vi "CRYMultitone Sine.vi"(0 "Start Freq":dbl, 1 "Fs":dbl, 2 "Level In":dbl, 5 "Stop Freq":dbl, 7 "Step Number":i32, 9 "Resolution":u16, 11 "Cycles":dbl=1.0 max=3.0 step=1.0, 12 "Freq Rounding":bool, 13 "Rounding value":dbl, 14 "FAPS In":T1(array[cluster])) -> (4 "FAPS Out":T1(array[cluster]))   [LabVIEW 2013]
uses:
  CRYStimulus Global.vi
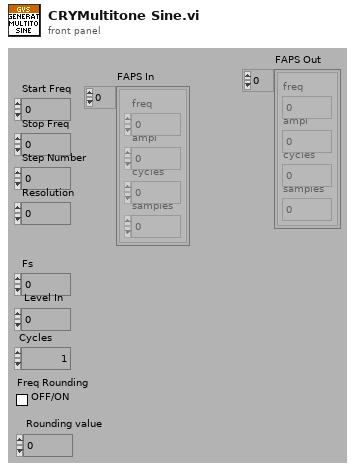
[diagram p1: front panel]
types:
  T1 = cluster{"freq":dbl, "ampl":dbl, "cycles":dbl, "samples":i32}[]
  T2 = cluster{"freq":dbl, "ampl":dbl, "cycles":dbl, "samples":i32}
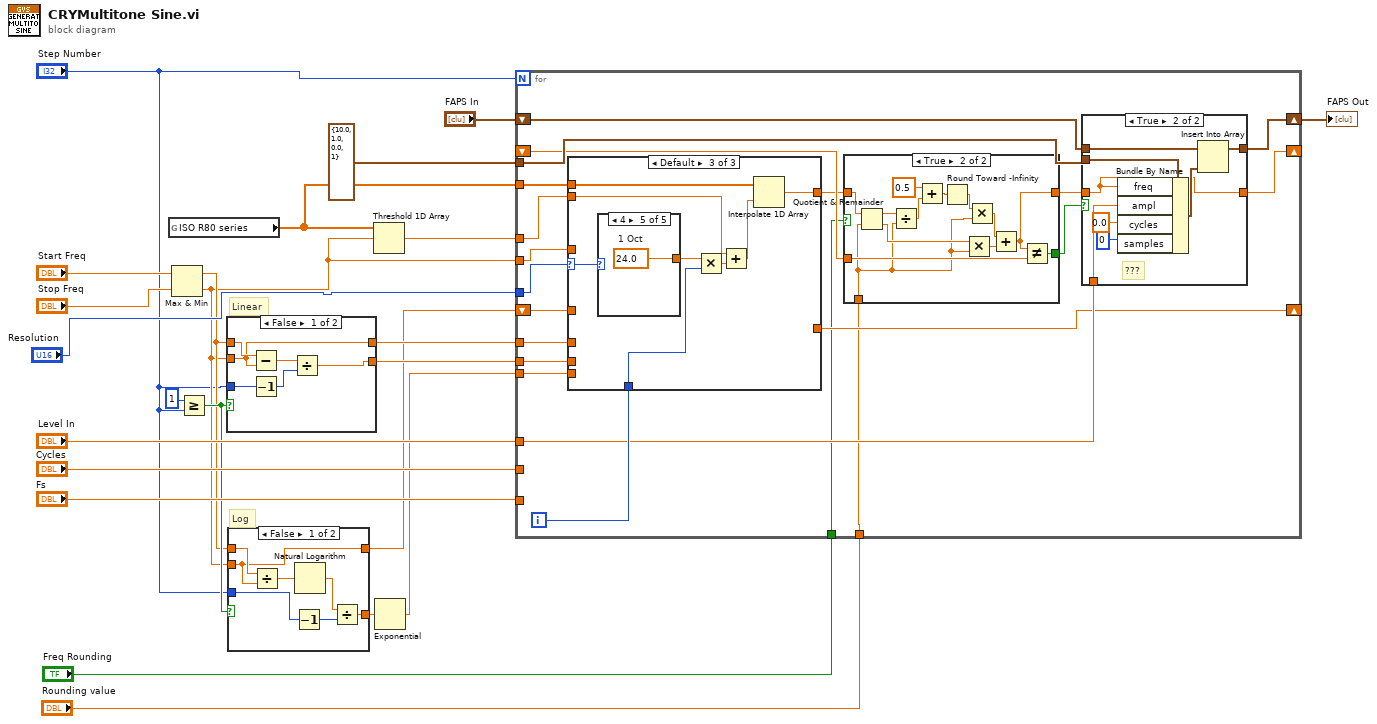
[diagram p0: block diagram]
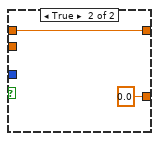
[diagram p2: hidden frame]
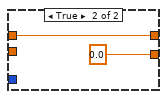
[diagram p3: hidden frame]
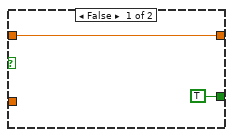
[diagram p4: hidden frame]
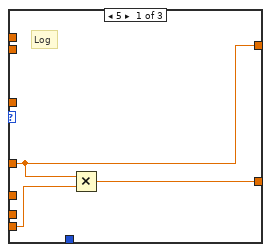
[diagram p6: hidden frame]
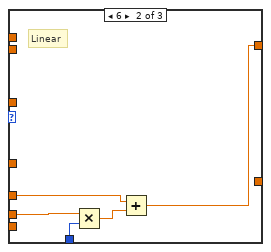
[diagram p7: hidden frame]
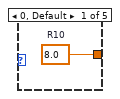
[diagram p8: hidden frame]
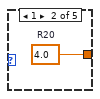
[diagram p9: hidden frame]
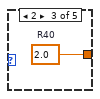
[diagram p10: hidden frame]
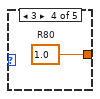
[diagram p11: hidden frame]
diagram:
  # "Linear"
  # "Log"
  n1 = global read "CRYStimulus Global.vi" "ISO R80 series"() -> (w1:dbl[])
  n2 = Max & Min(x="Start Freq", y="Stop Freq") -> (max(x,y)=w5:dbl, min(x,y)=w4:dbl)
  n3 = Greater Or Equal?(x=1, y="Step Number") -> (x >= y?=w6:bool)
  n4 = case shown="False" w6 {
    tunnel: w4 -> [w24 _]
    tunnel: [w24 w30] -> w14
    tunnel: [w25 0.0] -> w13
    tunnel: "Step Number" -> [w29 _]
    tunnel: w5 -> [w27 w30]
    frame False {
      n5 = Subtract(x=w27, y=w24) -> (x-y=w26:dbl)
      n6 = Decrement(x=w29) -> (x-1=w28:i32)
      n7 = Divide(x=w26, y=w28) -> (x/y=w25:dbl)
    }
    frame True {
    }
  }
  n8 = case shown="False" w6 {
    tunnel: w4 -> [w33 _]
    tunnel: w5 -> [w35 w40]
    tunnel: [w33 w40] -> w10
    tunnel: [w34 0.0] -> w12
    tunnel: "Step Number" -> [w32 _]
    frame False {
      n9 = Divide(x=w35, y=w33) -> (x/y=w38:dbl)
      n10 = Decrement(x=w32) -> (x-1=w36:i32)
      n11 = Natural Logarithm(1:w38) -> (0:w37:dbl)
      n12 = Divide(x=w37, y=w36) -> (x/y=w34:dbl)
    }
    frame True {
    }
  }
  n13 = Threshold 1D Array(2:w4, 3:w1) -> (0:w23:dbl)  [unwired: 1 out]
  n14 = Exponential(1:w12) -> (0:w11:dbl)
  n15 = for {
    N: "Step Number" -> [_]
    tunnel: w23 -> [w61]
    tunnel: T2 {"freq"=10.0, "ampl"=1.0, "cycles"=0.0, "samples"=1} -> [w60]
    shift-right: [w59] -> w16
    shift-left: "FAPS In" -> [w58]
    tunnel: "Resolution" -> [w54]
    tunnel: "Level In" -> [w56]
    tunnel: "Fs" -> [_]
    tunnel: "Cycles" -> [_]
    tunnel: w1 -> [w55]
    tunnel: w4 -> [w53]
    tunnel: w13 -> [w51]
    tunnel: w11 -> [w49]
    shift-right: [w48] -> _
    shift-left: w10 -> [w50]
    shift-right: [w41] -> _
    shift-left: _ -> [w47]
    tunnel: "Rounding value" -> [w46]
    tunnel: "Freq Rounding" -> [w44]
    tunnel: w14 -> [w52]
    i -> [w57]
    n16 = case shown="Default" w54 {
      selector: w54 -> [_ _ w95]
      tunnel: w61 -> [_ _ w102]
      tunnel: w57 -> [_ w93 w98]
      tunnel: [w88 w90 w97] -> w43
      tunnel: w55 -> [_ _ w96]
      tunnel: w53 -> [_ _ _]
      tunnel: w52 -> [_ w92 _]
      tunnel: w51 -> [_ w91 _]
      tunnel: w49 -> [w89 _ _]
      tunnel: w50 -> [w88 _ _]
      tunnel: [w87 _ _] -> w48
      frame 5 {
        # "Log"
        n17 = Multiply(x=w88, y=w89) -> (x*y=w87:dbl)
      }
      frame 6 {
        # "Linear"
        n18 = Multiply(x=w91, y=w93) -> (x*y=w94:dbl)
        n19 = Add(x=w92, y=w94) -> (x+y=w90:dbl)
      }
      frame Default {
        n20 = case shown="4" w95 {
          tunnel: [w103 w104 w105 w106 w107] -> w101
          frame 0, Default {
            w103 = 8.0  # R10
          }
          frame 1 {
            w104 = 4.0  # R20
          }
          frame 2 {
            w105 = 2.0  # R40
          }
          frame 3 {
            w106 = 1.0  # R80
          }
          frame 4 {
            w107 = 24.0  # 1 Oct
          }
        }
        n21 = Multiply(x=w101, y=w98) -> (x*y=w100:dbl)
        n22 = Add(x=w102, y=w100) -> (x+y=w99:dbl)
        n23 = Interpolate 1D Array(1:w99, 2:w96) -> (0:w97:dbl)
      }
    }
    n24 = case shown="True" w44 {
      tunnel: w47 -> [_ w74]
      tunnel: w46 -> [_ w67]
      tunnel: [TRUE w73] -> w45
      tunnel: [w63 w64] -> w42
      tunnel: w43 -> [w63 w65]
      frame False {
      }
      frame True {
        n25 = Quotient & Remainder(x=w65, y=w67) -> (x-y*floor(x/y)=w75:dbl, floor(x/y)=w72:dbl)
        n26 = Divide(x=w75, y=w67) -> (x/y=w68:dbl)
        n27 = Add(x=0.5, y=w68) -> (x+y=w70:dbl)
        n28 = Round Toward -Infinity(1:w70) -> (0:w66:dbl)
        n29 = Multiply(x=w72, y=w67) -> (x*y=w71:dbl)
        n30 = Multiply(x=w66, y=w67) -> (x*y=w76:dbl)
        n31 = Add(x=w76, y=w71) -> (x+y=w64:dbl)
        n32 = Not Equal?(x=w64, y=w74) -> (x != y?=w73:bool)
      }
    }
    n33 = case shown="True" w45 {
      tunnel: w60 -> [_ w86]
      tunnel: [w78 w85] -> w59
      tunnel: w58 -> [w78 w84]
      tunnel: w56 -> [_ w83]
      tunnel: w42 -> [w77 w79]
      tunnel: [w77 w79] -> w41
      frame False {
      }
      frame True {
        # "???"
        n34 = Bundle By Name(cluster=w86, "freq"=w79, "ampl"=w83, "cycles"=0.0 ("phase"), "samples"=0) -> (w81:T2)
        n35 = Insert Into Array(array=w84, new element=w81) -> (w85:T1)  [unwired: 1 in]
      }
    }
  }
  "FAPS Out" <- w16
